vi "MPXMessageLoop.vi"(8 "Error In":errorcluster, 11 "CommunicationRefs":T1) -> (0 "Error Out":errorcluster)   [LabVIEW 2015]
uses:
  TypeDefs/CommunicationRefs.ctl
  TypeDefs/MessageCluster.ctl
  TypeDefs/MPXSettings.ctl
  TypeDefs/MPXMicropump.ctl
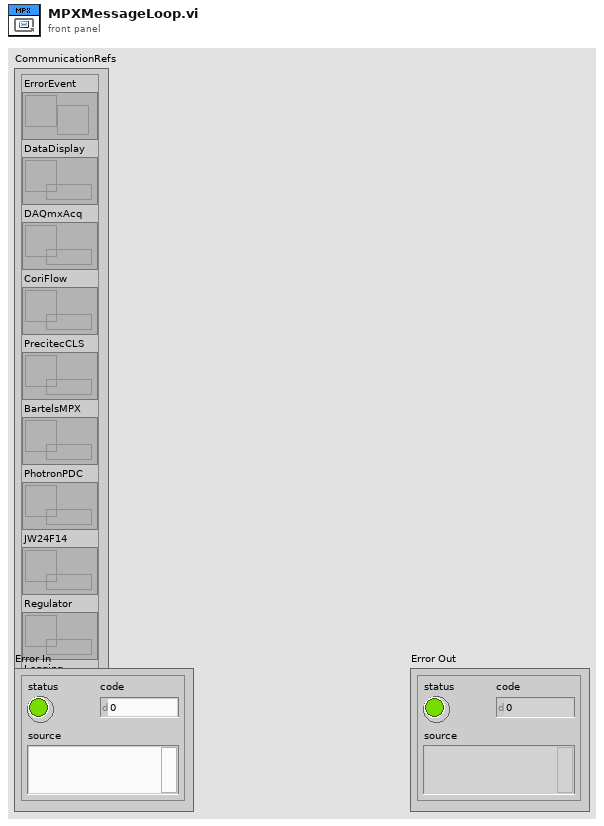
[diagram p1: front panel]
types:
  T1 = typedef "CommunicationRefs.ctl" = cluster{"ErrorEvent":refnum<user-event>, "DataDisplay":refnum<queue>, "DAQmxAcq":refnum<queue>, "CoriFlow":refnum<queue>, "PrecitecCLS":refnum<queue>, "BartelsMPX":refnum<queue>, "PhotronPDC":refnum<queue>, "JW24F14":refnum<queue>, "Regulator":refnum<queue>, "Logging":refnum<queue>}
  T2 = typedef "MPXSettings.ctl" = cluster{"MPX Port":refnum<visa-resource-name>, "Simulate":bool}
  T3 = typedef "MPXMicropump.ctl" = cluster{"Signal Form":u16, "Frequency [Hz]":i32, "Amplitude [V]":i32, "MPX [ON/OFF]":bool}
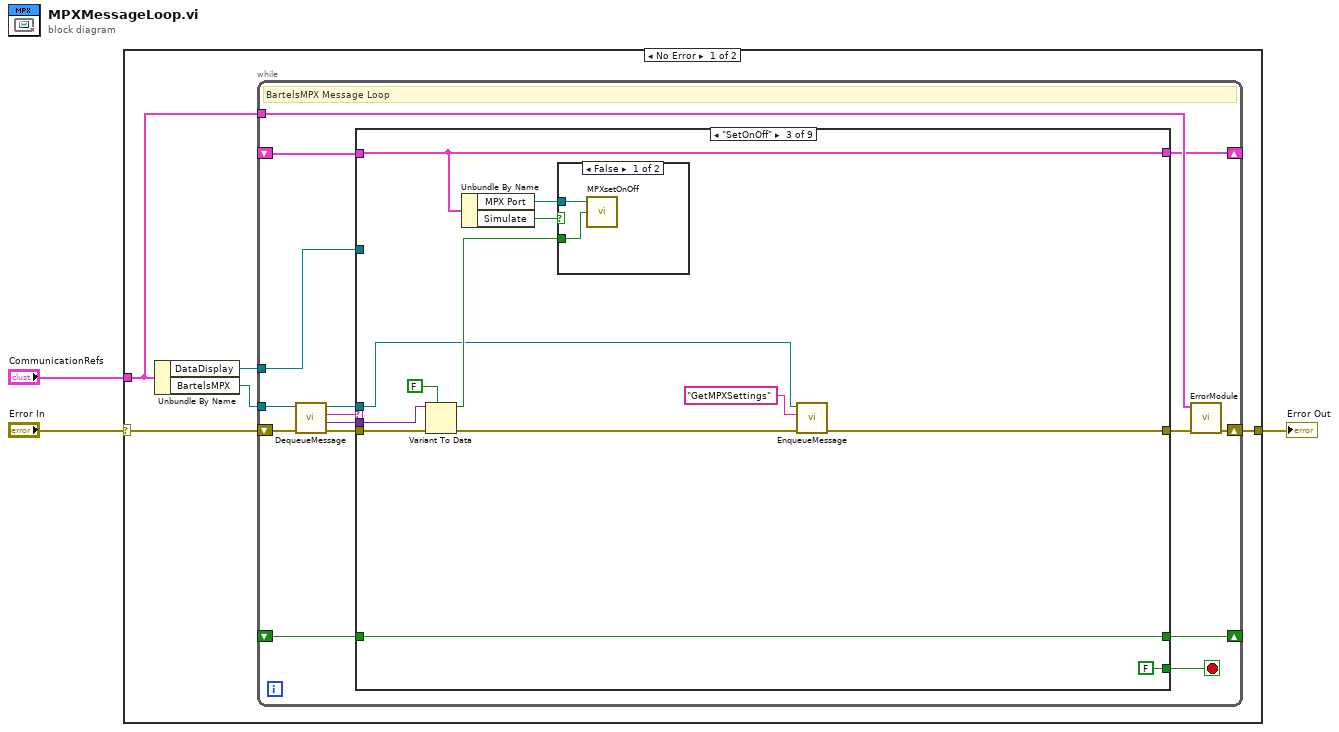
[diagram p0: block diagram]
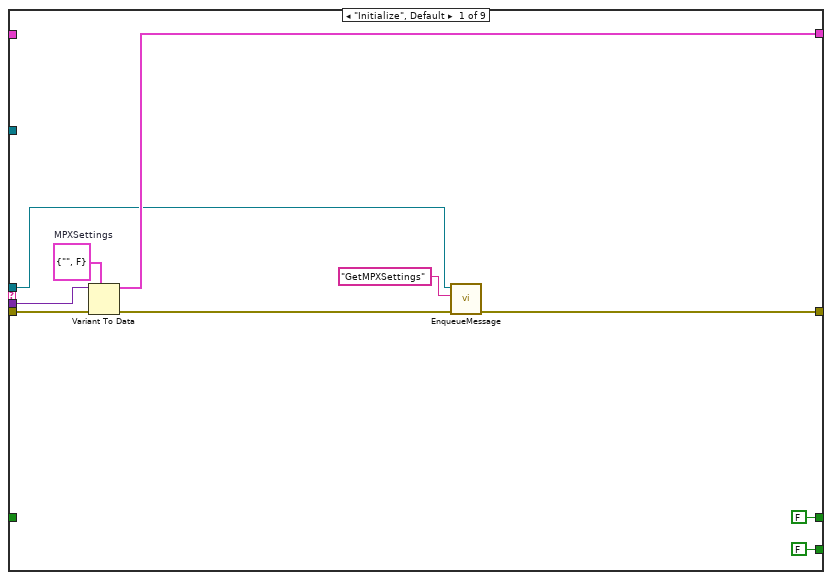
[diagram p2: hidden frame]
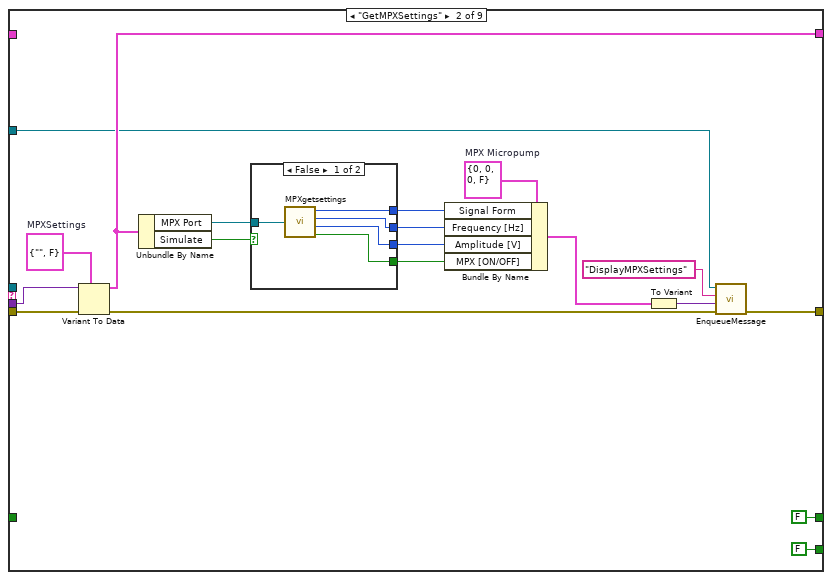
[diagram p3: hidden frame]
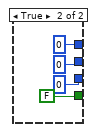
[diagram p4: hidden frame]
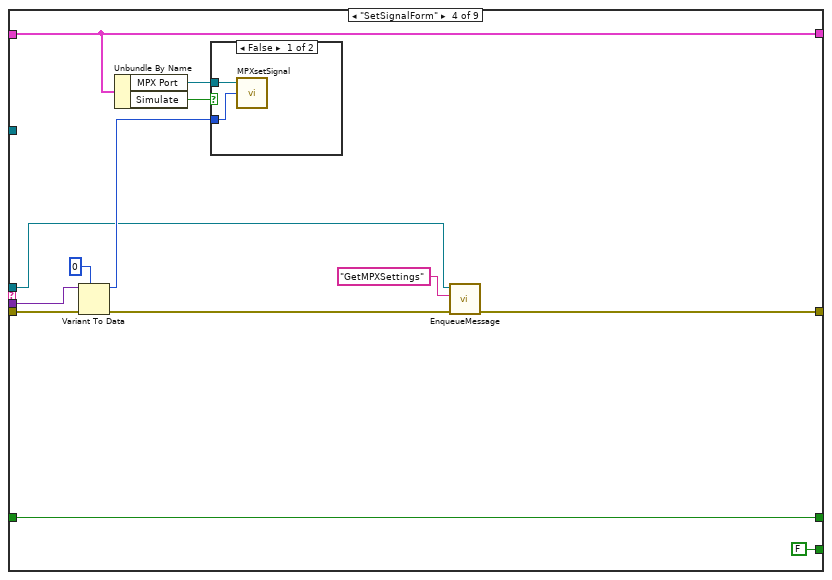
[diagram p6: hidden frame]
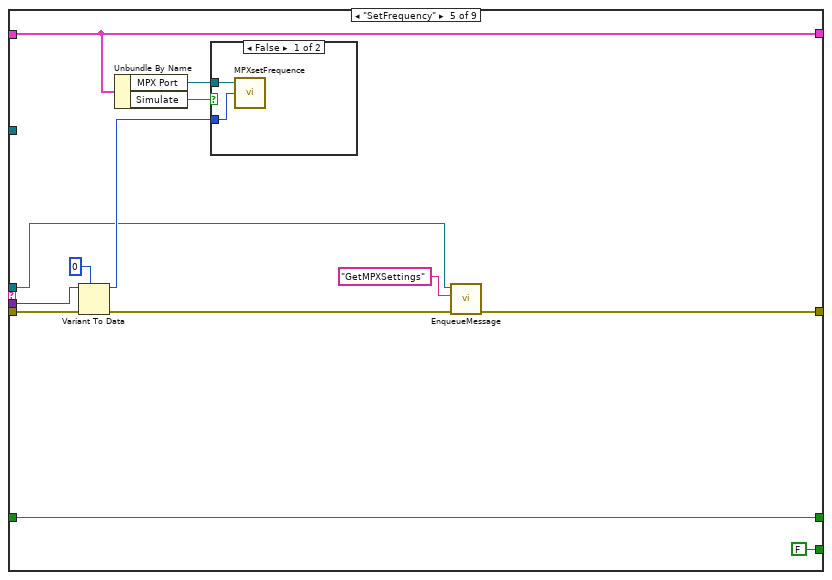
[diagram p8: hidden frame]
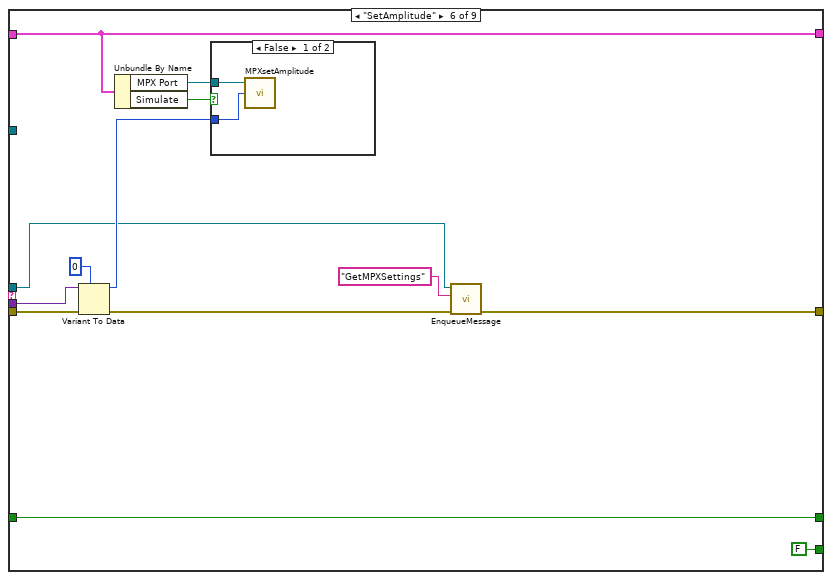
[diagram p10: hidden frame]
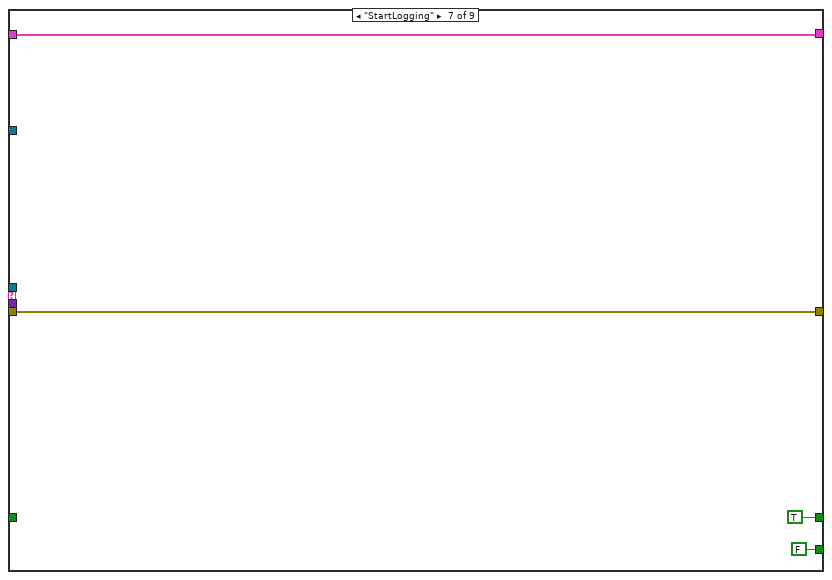
[diagram p12: hidden frame]
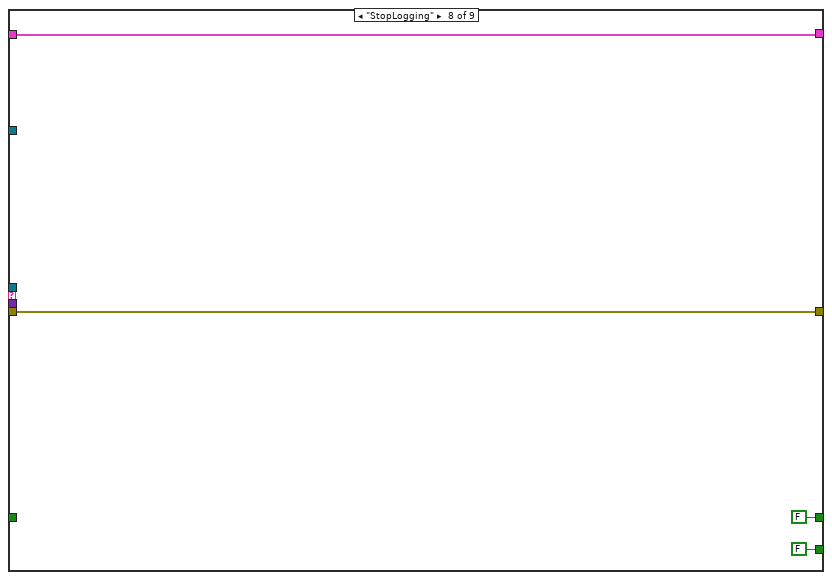
[diagram p13: hidden frame]
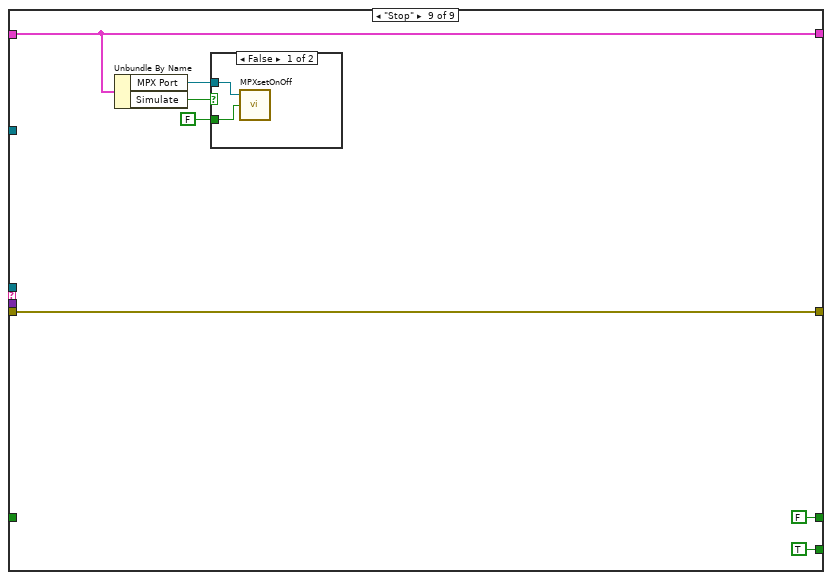
[diagram p14: hidden frame]
diagram:
  n1 = case shown="No Error" "Error In" {
    selector: "Error In" -> [w7 w139]
    tunnel: [w6 w139] -> w2
    tunnel: "CommunicationRefs" -> [w5 _]
    frame No Error {
      n2 = Unbundle By Name(w5) -> ("DataDisplay"=w4:refnum<queue>, "BartelsMPX"=w8:refnum<queue>)
      n3 = while {
        tunnel: w8 -> [w23]
        tunnel: w5 -> [w15]
        shift-right: [w17] -> w6
        shift-left: w7 -> [w22]
        shift-right: [w13] -> _
        shift-left: _ -> [w12]
        shift-right: [w11] -> _
        shift-left: _ -> [w10]
        tunnel: w4 -> [w9]
        stop <- w14 stop-if-true
        # "BartelsMPX Message Loop"
        n4 = call "DequeueMessage.vi"("error in (no error)"=w22, "MessageQueue"=w23) -> ("error out"=w18:errorcluster, "MessageData"=w19:variant, "Message"=w20:string, "dupMessageQueue"=w21:refnum<queue>)  [unwired: 6 in]
        n5 = case shown="\"SetOnOff\"" w20 {
          tunnel: w21 -> [w25 _ w62 w77 w92 w108 _ _ _]
          tunnel: w19 -> [w31 w50 w72 w87 w102 w117 _ _ _]
          tunnel: w18 -> [w32 w51 w73 w88 w103 w118 w124 w128 w135]
          tunnel: [w26 w43 w64 w79 w94 w109 w124 w128 w135] -> w16
          tunnel: [FALSE FALSE FALSE FALSE FALSE FALSE FALSE FALSE TRUE] -> w14
          tunnel: [w29 w48 w69 w84 w99 w114 w125 w129 w132] -> w13
          tunnel: w12 -> [_ _ w69 w84 w99 w114 w125 w129 w132]
          tunnel: [FALSE FALSE w66 w82 w97 w112 TRUE FALSE FALSE] -> w11
          tunnel: w10 -> [_ _ w66 w82 w97 w112 _ _ _]
          tunnel: w9 -> [_ w42 _ _ _ _ _ _ _]
          frame "Initialize", Default {
            w30 = T2 {"MPX Port"="", "Simulate"=FALSE}  # MPXSettings
            n6 = Variant To Data(error in=w32, type=w30, Variant=w31) -> (data=w29:T2, error out=w27:errorcluster)
            n7 = call "EnqueueMessage.vi"("error in (no error)"=w27, "Message"="GetMPXSettings", "MessageQueue"=w25) -> ("error out"=w26:errorcluster)  [unwired: 7 in, 1 out]
          }
          frame "GetMPXSettings" {
            w40 = T3 {"Signal Form"=0, "Frequency [Hz]"=0, "Amplitude [V]"=0, "MPX [ON/OFF]"=FALSE}  # MPX Micropump
            w49 = T2 {"MPX Port"="", "Simulate"=FALSE}  # MPXSettings
            n8 = Variant To Data(error in=w51, type=w49, Variant=w50) -> (data=w48:T2, error out=w44:errorcluster)
            n9 = Unbundle By Name(w48) -> ("MPX Port"=w47:refnum<visa-resource-name>, "Simulate"=w46:bool)
            n10 = case shown="False" w46 {
              tunnel: w47 -> [w57 _]
              tunnel: [w56 u16 0 ("Waveform")] -> w39
              tunnel: [w55 0 ("Frequence [Hz]")] -> w38
              tunnel: [w54 0 ("Amplitude [V]")] -> w37
              tunnel: [w53 FALSE ("Signal On")] -> w36
              frame False {
                n11 = call "MPXgetsettings.vi"("VISA resource name"=w57) -> ("Signal On"=w53:bool, "Amplitude [V]"=w54:i32, "Frequence [Hz]"=w55:i32, "Waveform"=w56:u16)  [unwired: 1 out]
              }
              frame True {
              }
            }
            n12 = Bundle By Name(cluster=w40, "Signal Form"=w39, "Frequency [Hz]"=w38, "Amplitude [V]"=w37, "MPX [ON/OFF]"=w36) -> (w34:T3)
            n13 = To Variant(anything=w34) -> (Variant=w35:variant)
            n14 = call "EnqueueMessage.vi"("error in (no error)"=w44, "MessageData"=w35, "Message"="DisplayMPXSettings", "MessageQueue"=w42) -> ("error out"=w43:errorcluster)  [unwired: 6 in, 1 out]
          }
          frame "SetOnOff" {
            n15 = Variant To Data(error in=w73, type=FALSE, Variant=w72) -> (data=w67:bool, error out=w63:errorcluster)
            n16 = Unbundle By Name(w69) -> ("MPX Port"=w71:refnum<visa-resource-name>, "Simulate"=w70:bool)
            n17 = case shown="False" w70 {
              tunnel: w71 -> [w76 _]
              tunnel: w67 -> [w75 _]
              frame False {
                n18 = call "MPXsetOnOff.vi"("Signal On"=w75, "Comport in"=w76) -> ()  [unwired: 1 in, 2 out]
              }
              frame True {
              }
            }
            n19 = call "EnqueueMessage.vi"("error in (no error)"=w63, "Message"="GetMPXSettings", "MessageQueue"=w62) -> ("error out"=w64:errorcluster)  [unwired: 7 in, 1 out]
          }
          frame "SetSignalForm" {
            n20 = Variant To Data(error in=w88, type=u16 0 ("NewVal"), Variant=w87) -> (data=w83:u16, error out=w78:errorcluster)
            n21 = Unbundle By Name(w84) -> ("MPX Port"=w86:refnum<visa-resource-name>, "Simulate"=w85:bool)
            n22 = case shown="False" w85 {
              tunnel: w86 -> [w91 _]
              tunnel: w83 -> [w90 _]
              frame False {
                n23 = call "MPXsetSignal.vi"("Waveform"=w90, "Comport in"=w91) -> ()  [unwired: 1 in, 2 out]
              }
              frame True {
              }
            }
            n24 = call "EnqueueMessage.vi"("error in (no error)"=w78, "Message"="GetMPXSettings", "MessageQueue"=w77) -> ("error out"=w79:errorcluster)  [unwired: 7 in, 1 out]
          }
          frame "SetFrequency" {
            n25 = Variant To Data(error in=w103, type=0 ("NewVal"), Variant=w102) -> (data=w98:i32, error out=w93:errorcluster)
            n26 = Unbundle By Name(w99) -> ("MPX Port"=w101:refnum<visa-resource-name>, "Simulate"=w100:bool)
            n27 = case shown="False" w100 {
              tunnel: w101 -> [w106 _]
              tunnel: w98 -> [w105 _]
              frame False {
                n28 = call "MPXsetFrequence.vi"("Frequence [Hz]"=w105, "Comport in"=w106) -> ()  [unwired: 1 in, 2 out]
              }
              frame True {
              }
            }
            n29 = call "EnqueueMessage.vi"("error in (no error)"=w93, "Message"="GetMPXSettings", "MessageQueue"=w92) -> ("error out"=w94:errorcluster)  [unwired: 7 in, 1 out]
          }
          frame "SetAmplitude" {
            n30 = Variant To Data(error in=w118, type=0 ("NewVal"), Variant=w117) -> (data=w113:i32, error out=w107:errorcluster)
            n31 = Unbundle By Name(w114) -> ("MPX Port"=w116:refnum<visa-resource-name>, "Simulate"=w115:bool)
            n32 = case shown="False" w115 {
              tunnel: w116 -> [w121 _]
              tunnel: w113 -> [w120 _]
              frame False {
                n33 = call "MPXsetAmplitude.vi"("Amplitude [V]"=w120, "Comport in"=w121) -> ()  [unwired: 1 in, 2 out]
              }
              frame True {
              }
            }
            n34 = call "EnqueueMessage.vi"("error in (no error)"=w107, "Message"="GetMPXSettings", "MessageQueue"=w108) -> ("error out"=w109:errorcluster)  [unwired: 7 in, 1 out]
          }
          frame "StartLogging" {
          }
          frame "StopLogging" {
          }
          frame "Stop" {
            n35 = Unbundle By Name(w132) -> ("MPX Port"=w134:refnum<visa-resource-name>, "Simulate"=w133:bool)
            n36 = case shown="False" w133 {
              tunnel: w134 -> [w138 _]
              tunnel: FALSE -> [w137 _]
              frame False {
                n37 = call "MPXsetOnOff.vi"("Signal On"=w137, "Comport in"=w138) -> ()  [unwired: 1 in, 2 out]
              }
              frame True {
              }
            }
          }
        }
        n38 = call "ErrorModule.vi"("Error In"=w16, "CommunicationRefs"=w15) -> ("Error Out"=w17:errorcluster)  [unwired: 9 in]
      }
    }
    frame Error {
    }
  }
  "Error Out" <- w2
